vi "auto_angle.vi"(8 "column":i32, 9 "row":i32, 10 "element":T1=255, 11 "pieceOfWorld in":T2[][](array[typedef])) -> (2 "found?":bool, 3 "angle":dbl)   [LabVIEW 2015, in "PolyVIEW.lvclass"]
uses:
  PolyVIEW.lvclass
  actors/world/typedefs/worldCell_cluster.ctl
  actors/world/typedefs/markValue_cluster.ctl
  actors/world/typedefs/markValue.ctl
  actors/world/typedefs/markVolume.ctl
  actors/world/typedefs/amountOfFood.ctl
  actors/world/typedefs/anthillType_enum.ctl
  actors/world/world.lvlib
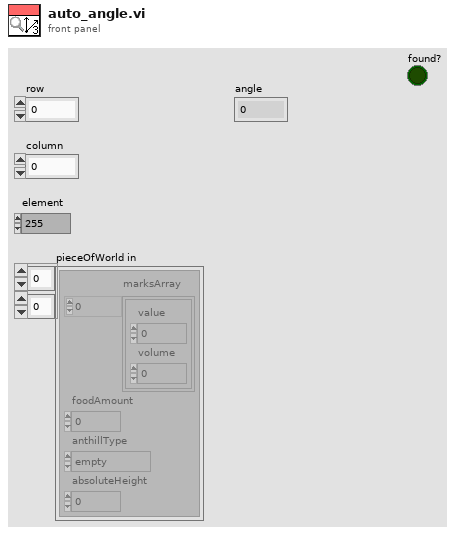
[diagram p1: front panel]
types:
  T1 = typedef "world.lvlib/markValue.ctl" = u8
  T2 = typedef "world.lvlib/worldCell_cluster.ctl" = cluster{"marksArray":T3[], "foodAmount":T5, "anthillType":T6, "absoluteHeight":u8}
  T3 = typedef "world.lvlib/markValue_cluster.ctl" = cluster{"value":T1, "volume":T4}
  T4 = typedef "world.lvlib/markVolume.ctl" = u16
  T5 = typedef "world.lvlib/amountOfFood.ctl" = i32
  T6 = typedef "world.lvlib/anthillType_enum.ctl" = enum16{"empty", "own", "rival"}
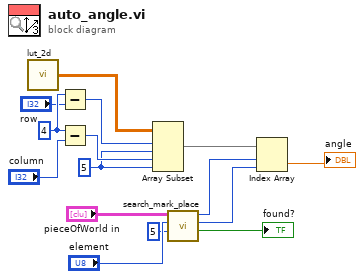
[diagram p0: block diagram]
diagram:
  w13 = 4
  w9 = 5 ("length")
  n1 = call "lut_2d.vi"() -> ("output array"=w7:dbl[][])
  n2 = Subtract(x=w13, y="row") -> (x-y=w11:i32)
  n3 = Subtract(x=w13, y="column") -> (x-y=w14:i32)
  n4 = Array Subset(array=w7, index (row)=w11, length (row)=w9, index (col)=w14, length (col)=w9) -> (w8:dbl[][])
  n5 = call "search_mark_place.vi"("square"=5, "element"="element", "pieceOfWorld in"="pieceOfWorld in") -> ("found?"=→"found?":bool, "column"=w4:i32, "row"=w3:i32)  [unwired: 5 in, 1 out]
  n6 = Index Array(array=w8, index (row)=w3, index (col)=w4) -> (element=→"angle":dbl)
